vi "setParameters.vi"(10 "Parameters":T1, 11 "StandbyCommand in":refnum<class "StandbyCommand.lvclass">) -> (3 "StandbyCommand out":refnum<class "StandbyCommand.lvclass">)   [LabVIEW 2016, in "StandbyCommand.lvclass"]
uses:
  StandbyCommand.lvclass
  DataTypes/Topics/CommandStandby.ctl
  DataTypes/Topics/Parts/CommandId.ctl
  StandbyCommand.lvclass/StandbyCommand.ctl
  DataTypes/Topics/M1M3SupportTopics.lvlib
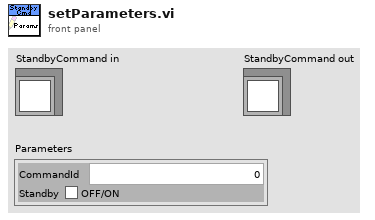
[diagram p1: front panel]
types:
  T1 = typedef "M1M3SupportTopics.lvlib/CommandStandby.ctl" = cluster{"CommandId":T2, "Standby":bool}
  T2 = typedef "M1M3SupportTopics.lvlib/CommandId.ctl" = i32
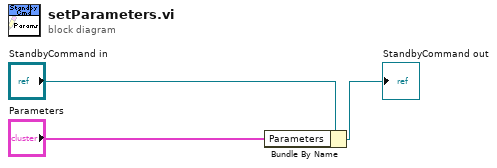
[diagram p0: block diagram]
diagram:
  n1 = Bundle By Name(cluster="StandbyCommand in", "Parameters"="Parameters") -> (→"StandbyCommand out":refnum<class "StandbyCommand.lvclass">)
